vi "test_Monitor Data Queue.vi"(8 "error in (no error)":errorcluster) -> (0 "error out":errorcluster, 3 "Passed?":bool)   [LabVIEW 2016]
uses:
  Host/Typedefs/Monitor Data Operation.ctl
  Host/Typedefs/Monitor Data Element.ctl
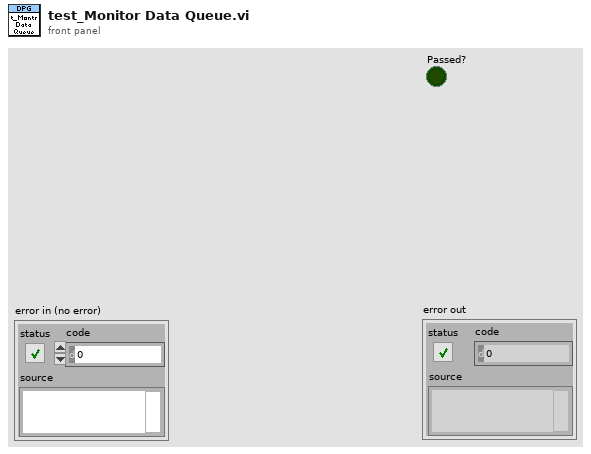
[diagram p1: front panel]
types:
  T1 = typedef "Monitor Data Element.ctl" = cluster{"Pin Data":u32, "Transition ":u32}
  T2 = typedef "Monitor Data Operation.ctl" = enum16{"Obtain", "Enqueue", "Read Elements", "Flush", "Release", "Read Last Element"}
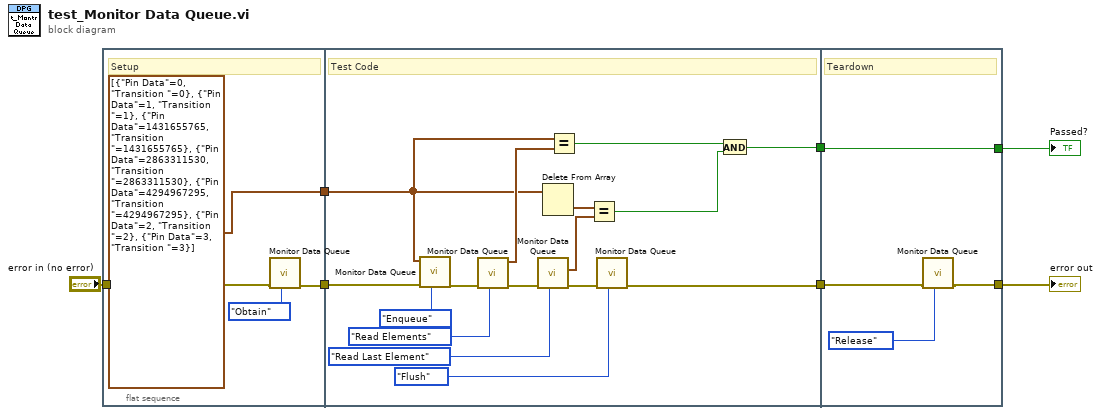
[diagram p0: block diagram]
diagram:
  n1 = flat-sequence {
    tunnel: "error in (no error)" -> [w11]
    tunnel: [w10] -> w7
    tunnel: [T1[] [{"Pin Data"=0, "Transition "=0}, {"Pin Data"=1, "Transition "=1}, {"Pin Data"=1431655765, "Transition "=1431655765}, {"Pin Data"=2863311530, "Transition "=2863311530}, {"Pin Data"=4294967295, "Transition "=4294967295}, {"Pin Data"=2, "Transition "=2}, {"Pin Data"=3, "Transition "=3}] ("Data From FIFO")] -> w1
    tunnel: w7 -> [w26]
    tunnel: [w18] -> w4
    tunnel: [w27] -> w3
    tunnel: w1 -> [w13]
    tunnel: [w30] -> w5
    tunnel: w4 -> [w31]
    tunnel: w3 -> [w28]
    tunnel: [w28] -> w2
    frame #0 {
      # "Setup"
      n2 = call "Monitor Data Queue.vi"("Queue Function"=Monitor_Data_Operation."Obtain", "error in (no error)"=w11) -> ("error out"=w10:errorcluster)  [unwired: 6 in, 3 out]
    }
    frame #1 {
      # "Test Code"
      n3 = call "Monitor Data Queue.vi"("Queue Function"=Monitor_Data_Operation."Enqueue", "error in (no error)"=w26, "Data From FIFO"=w13) -> ("error out"=w24:errorcluster)  [unwired: 5 in, 3 out]
      n4 = call "Monitor Data Queue.vi"("Queue Function"=Monitor_Data_Operation."Read Elements", "error in (no error)"=w24) -> ("error out"=w22:errorcluster, "Queue Elements"=w17:T1[])  [unwired: 6 in, 2 out]
      n5 = call "Monitor Data Queue.vi"("Queue Function"=Monitor_Data_Operation."Read Last Element", "error in (no error)"=w22) -> ("error out"=w20:errorcluster, "Last Queue Element"=w16:T1)  [unwired: 6 in, 2 out]
      n6 = Delete From Array(array=w13) -> (deleted portion=w15:T1)  [unwired: 2 in, 1 out]
      n7 = Equal?(x=w13, y=w17) -> (x = y?=w12:bool)
      n8 = Equal?(x=w15, y=w16) -> (x = y?=w14:bool)
      n9 = call "Monitor Data Queue.vi"("Queue Function"=Monitor_Data_Operation."Flush", "error in (no error)"=w20) -> ("error out"=w18:errorcluster)  [unwired: 6 in, 3 out]
      n10 = And(x=w12, y=w14) -> (x .and. y?=w27:bool)
    }
    frame #2 {
      # "Teardown"
      n11 = call "Monitor Data Queue.vi"("Queue Function"=Monitor_Data_Operation."Release", "error in (no error)"=w31) -> ("error out"=w30:errorcluster)  [unwired: 6 in, 3 out]
    }
  }
  "error out" <- w5
  "Passed?" <- w2
